vi "VeriStand Web Service Demo.Async.vi"(10 "Parameters":variant, 11 "Process":refnum<class "Process.lvclass">) -> ()   [LabVIEW 2017, in "VeriStand Web Service Demo Engine.lvlib"]
uses:
  VeriStand Web Service Demo Engine.lvlib
  <vilib>/NI/NIVS Inline Async API/_VS Inline Async API/Process/Process.lvclass
  Shared/Compiled.Settings.ctl
  <vilib>/NI/NIVS Inline Async API/_VS Inline Async API/Process/Process.lvclass/Process.ctl
  <vilib>/NI/NIVS Inline Async API/_Data Access Engine/Access Type Classes/Read/Read.lvclass/Read.ctl
  <vilib>/NI/NIVS Inline Async API/_Data Access Engine/Access Type Classes/Write/Write.lvclass/Write.ctl
  <vilib>/NI/NIVS Inline Async API/_Data Access Engine/Data Access Engine/Methods/Read.Data.vi
  <vilib>/NI/NIVS Inline Async API/_Data Access Engine/Data Access Engine/Methods/Write.Data.vi
  <vilib>/NI/NIVS Inline Async API/_VS Inline Async API/Process/Data Member Access/Read Data Access.vi
  <vilib>/NI/NIVS Inline Async API/_VS Inline Async API/Error Handling Process/SubVIs/Error.ConvertArray.vi
  <vilib>/NI/NIVS Inline Async API/_Data Access Engine/Access Type Classes/Read/Read.ProcessData.vi
  <vilib>/NI/NIVS Inline Async API/_Data Access Engine/Access Type Classes/Write/Write.ProcessData.vi
  <vilib>/NI/NIVS Inline Async API/_Data Access Engine/Data Access Engine/Methods/Read.Lookup.vi
  <vilib>/NI/NIVS Inline Async API/_Data Access Engine/Data Access Engine/Methods/Write.Lookup.vi
  <vilib>/NI/NIVS Inline Async API/_Data Access Engine/Data Access Engine/Data Access Engine.lvclass
  <vilib>/NI/VeriStand Web Service/vsws_api/vsws.lvlib
  Shared/VeriStand Web Service Demo Shared.lvlib
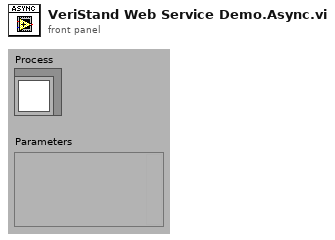
[diagram p1: front panel]
types:
  T1 = typedef "VeriStand Web Service Demo Shared.lvlib/Compiled.Settings.ctl" = cluster{"queueName":string}
  T2 = typedef "Data Access Engine.lvlib/Data Access Engine.lvclass/Write.DVR.ctl" = refnum<data-value>
  T3 = typedef "Data Access Engine.lvlib/Data Access Engine.lvclass/Read.DVR.ctl" = refnum<data-value>
  T4 = typedef "vsws.lvlib/cmdRef.ctl" = cluster{"queueRef":refnum<queue>, "reponseQueue":refnum<queue>}
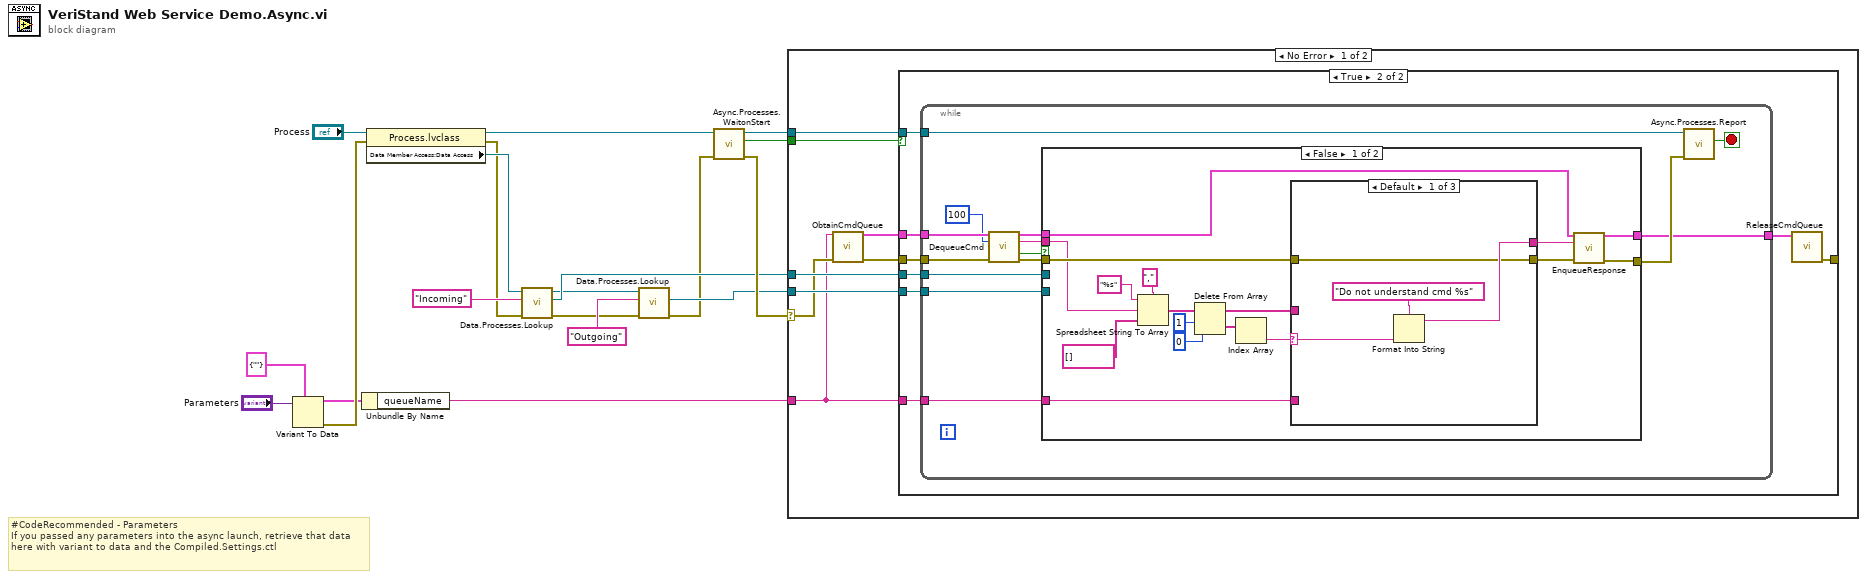
[diagram p0: block diagram]
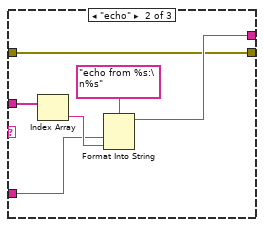
[diagram p3: hidden frame]
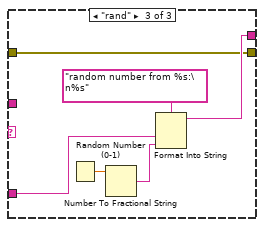
[diagram p4: hidden frame]
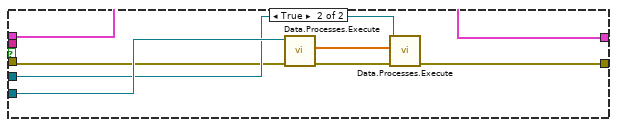
[diagram p5: hidden frame]
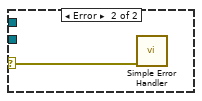
[diagram p6: hidden frame]
diagram:
  # "#CodeRecommended - Parameters\nIf you passed any parameters into the async launch, retrieve that data here with variant to data and the Compiled.Settings.ctl"
  n1 = Variant To Data(type=T1 {"queueName"=""} ("Compiled.Settings"), Variant="Parameters") -> (data=w2:T1, error out=w3:errorcluster)  [unwired: 1 in]
  n2 = Unbundle By Name(w2) -> ("queueName"=w1:string)
  n3 = property class="Process.lvclass"(reference="Process", error in=w3) -> (reference out=w8:refnum<class "Process.lvclass">, error out=w6:errorcluster, "Data Member Access:Data Access"=w7:refnum<class "Data Access Engine.lvclass">)
  n4 = call-poly <vilib>:"Data.Processes.Lookup.vi"("error in (no error)"=w6, "Name"="Incoming", "Data Access API in"=w7) -> ("error out"=w13:errorcluster, "Ref"=w12:T2, "Data Access API out"=w11:refnum<class "Data Access Engine.lvclass">)  [unwired: 5 in, 1 out]
  n5 = call-poly <vilib>:"Data.Processes.Lookup.vi"("error in (no error)"=w13, "Name"="Outgoing", "Data Access API in"=w11) -> ("error out"=w10:errorcluster, "Ref"=w15:T3)  [unwired: 5 in, 2 out]
  n6 = call <vilib>:"Async.Processes.WaitonStart.vi"("error in (no error)"=w10, "Process"=w8) -> ("error out"=w17:errorcluster, "Execute"=w19:bool, "Process out"=w18:refnum<class "Process.lvclass">)  [unwired: 7 in]
  n7 = case shown="No Error" w17 {
    selector: w17 -> [w23 w91]
    tunnel: w19 -> [w27 _]
    tunnel: w18 -> [w26 _]
    tunnel: w12 -> [w25 _]
    tunnel: w15 -> [w24 _]
    tunnel: w1 -> [w20 _]
    frame No Error {
      n8 = call <vilib>:"ObtainCmdQueue.vi"("queueName"=w20, "error in (no error)"=w23) -> ("cmdRef"=w21:T4, "error out"=w22:errorcluster)  [unwired: 12 in]
      n9 = case shown="True" w27 {
        tunnel: w22 -> [w28 w33]
        tunnel: w26 -> [_ w34]
        tunnel: w24 -> [_ w36]
        tunnel: w25 -> [_ w35]
        tunnel: w21 -> [_ w32]
        tunnel: w20 -> [_ w31]
        tunnel: [w28 w29] -> _
        frame False {
        }
        frame True {
          n10 = while {
            tunnel: w33 -> [w44]
            tunnel: w34 -> [w50]
            tunnel: w36 -> [w48]
            tunnel: w35 -> [w47]
            tunnel: w32 -> [w45]
            tunnel: w31 -> [w38]
            tunnel: [w37] -> w30
            stop <- w49 stop-if-true
            n11 = call <vilib>:"DequeueCmd.vi"("cmdRef in"=w45, "timeout in ms (-1)"=100 ("timeout ms"), "error in (no error)"=w44) -> ("cmdRef out"=w40:T4, "postdata"=w39:string, "timed out?"=w41:bool, "error out"=w43:errorcluster)  [unwired: 9 in]
            n12 = case shown="False" w41 {
              tunnel: w48 -> [_ w90]
              tunnel: w47 -> [_ w89]
              tunnel: [w54 w86] -> w46
              tunnel: w43 -> [w63 w85]
              tunnel: w40 -> [w64 w84]
              tunnel: w39 -> [w51 _]
              tunnel: w38 -> [w57 _]
              tunnel: [w53 w84] -> w37
              frame False {
                n13 = Spreadsheet String To Array(delimiter (Tab)=",", format string="%s" ("spreadsheet string"), spreadsheet string=w51, array type (2D Dbl)=string[] []) -> (array=w65:string[])
                n14 = Delete From Array(array=w65, length=1, index=0) -> (deleted portion=w59:string[], array with subset deleted=w60:string[])
                n15 = Index Array(array=w59) -> (element=w58:string)  [unwired: 1 in]
                n16 = case shown="Default" w58 {
                  selector: w58 -> [w70 _ _]
                  tunnel: w63 -> [w68 w72 w78]
                  tunnel: w60 -> [_ w77 _]
                  tunnel: w57 -> [_ w74 w82]
                  tunnel: [w69 w73 w79] -> w56
                  tunnel: [w68 w72 w78] -> w55
                  frame Default {
                    n17 = Format Into String(format string="Do not understand cmd %s", w70) -> (resulting string=w69:string)  [unwired: 2 in, 1 out]
                  }
                  frame "echo" {
                    n18 = Index Array(array=w77) -> (element=w75:string)  [unwired: 1 in]
                    n19 = Format Into String(format string="echo from %s:\n%s", w74, w75) -> (resulting string=w73:string)  [unwired: 2 in, 1 out]
                  }
                  frame "rand" {
                    n20 = Random Number (0-1)() -> (number: 0 to 1=w81:dbl)
                    n21 = Number To Fractional String(number=w81) -> (F-format string=w80:string)  [unwired: 3 in]
                    n22 = Format Into String(format string="random number from %s:\n%s", w82, w80) -> (resulting string=w79:string)  [unwired: 2 in, 1 out]
                  }
                }
                n23 = call <vilib>:"EnqueueResponse.vi"("cmdRef in"=w64, "response"=w56, "error in (no error)"=w55) -> ("cmdRef out"=w53:T4, "error out"=w54:errorcluster)  [unwired: 11 in]
              }
              frame True {
                n24 = call-poly <vilib>:"Data.Processes.Execute.vi"("error in (no error)"=w85, "Ref"=w90) -> ("error out"=w88:errorcluster, "Values"=w87:dbl[])  [unwired: 7 in, 1 out]
                n25 = call-poly <vilib>:"Data.Processes.Execute.vi"("error in (no error)"=w88, "Values"=w87, "Ref"=w89) -> ("error out"=w86:errorcluster)  [unwired: 8 in]
              }
            }
            n26 = call <vilib>:"Async.Processes.Report.vi"("Error"=w46, "Process in"=w50) -> ("Stop"=w49:bool)  [unwired: 8 in, 1 out]
          }
          n27 = call <vilib>:"ReleaseCmdQueue.vi"("cmdRef"=w30) -> ("error out"=w29:errorcluster)  [unwired: 14 in]
        }
      }
    }
    frame Error {
      n28 = call <vilib>:"Simple Error Handler.vi"("error in (no error)"=w91) -> ()  [unwired: 4 in, 5 out]
    }
  }
